vi "Stop.vi"(8 "error in (no error)":errorcluster, 11 "Electrophysiology in":refnum<class "AcquireTraces.lvclass">) -> (0 "error out":errorcluster, 3 "Electrophysiology out":refnum<class "AcquireTraces.lvclass">)   [LabVIEW 2010, in "AcquireTraces.lvclass"]
uses:
  AcquireTraces.lvclass
  AcquireTraces.lvclass/AcquireTraces.ctl
  Z:/libraries/HDF5Tools/LabView/HDF5Tools.lvlib
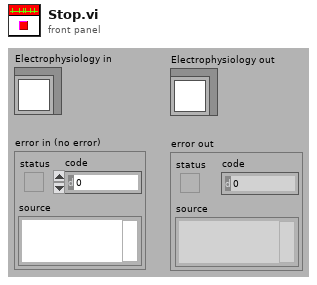
[diagram p1: front panel]
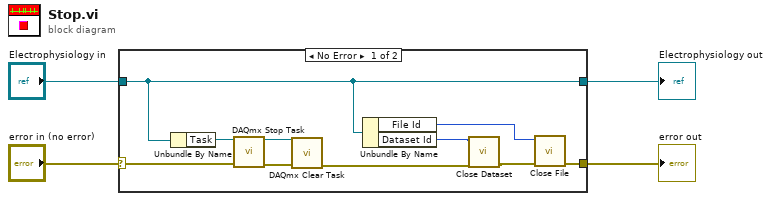
[diagram p0: block diagram]
diagram:
  n1 = case shown="No Error" "error in (no error)" {
    selector: "error in (no error)" -> [w11 w16]
    tunnel: [w6 w16] -> w3
    tunnel: [w10 w15] -> w1
    tunnel: "Electrophysiology in" -> [w10 w15]
    frame No Error {
      n2 = Unbundle By Name(w10) -> ("Task"=w12:refnum<k21>)
      n3 = call <vilib>:"DAQmx Stop Task.vi"("task/channels in"=w12, "error in"=w11) -> ("task out"=w14:refnum<k21>, "error out"=w13:errorcluster)  [unwired: 12 in]
      n4 = call <vilib>:"DAQmx Clear Task.vi"("task in"=w14, "error in"=w13) -> ("error out"=w5:errorcluster)  [unwired: 13 in]
      n5 = Unbundle By Name(w10) -> ("File Id"=w9:u64, "Dataset Id"=w8:u64)
      n6 = call "Close Dataset.vi"("error in (no error)"=w5, "dataset_id"=w8) -> ("error out"=w7:errorcluster)  [unwired: 9 in]
      n7 = call "Close File.vi"("error in (no error)"=w7, "file_id"=w9) -> ("error out"=w6:errorcluster)  [unwired: 9 in]
    }
    frame Error {
    }
  }
  "error out" <- w3
  "Electrophysiology out" <- w1
